vi "RF_Synth_init.vi"(1 "Initialize Instrument":u64, 2 "Inst_param":T1) -> ()   [LabVIEW 2013]
panel:
  out "Command out":string
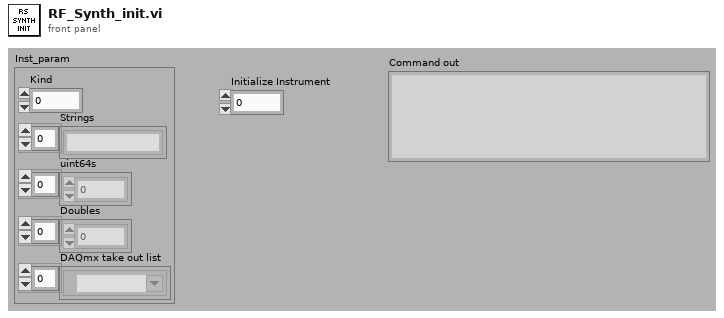
[diagram p1: front panel]
types:
  T1 = cluster{"Kind":u16, "Strings":string[], "uint64s":u64[], "Doubles":dbl[], "DAQmx take out list":refnum<k21>[]}
  T2 = enum16{"Frequency (GHz)", "Power (dBm)", "Phase (deg)", "Output on?", "Trigger mode", "Set channel", "Init"}[]
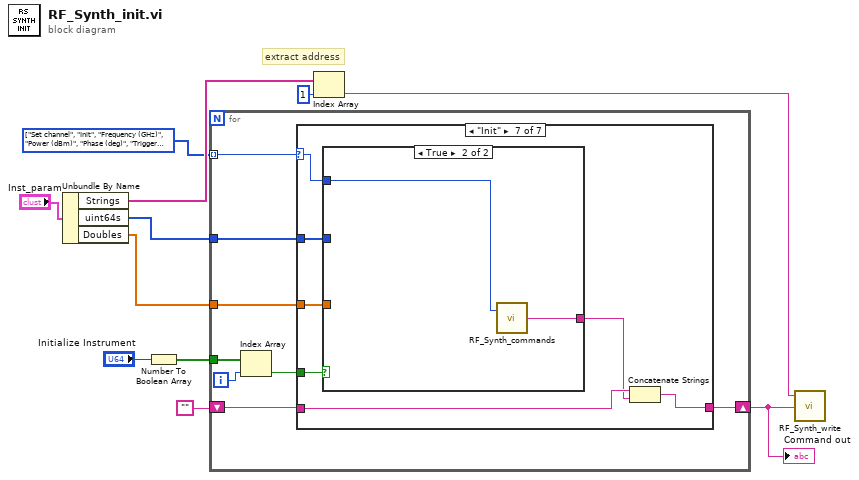
[diagram p0: block diagram]
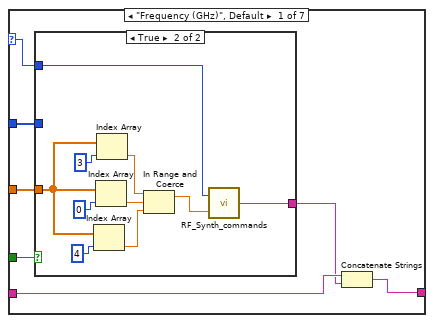
[diagram p2: hidden frame]
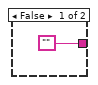
[diagram p3: hidden frame]
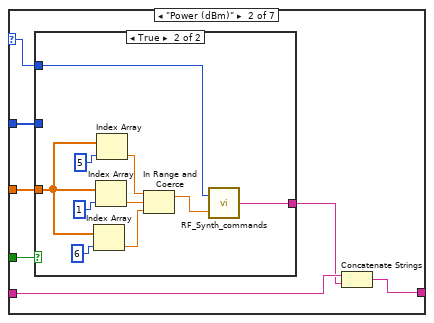
[diagram p4: hidden frame]
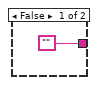
[diagram p5: hidden frame]
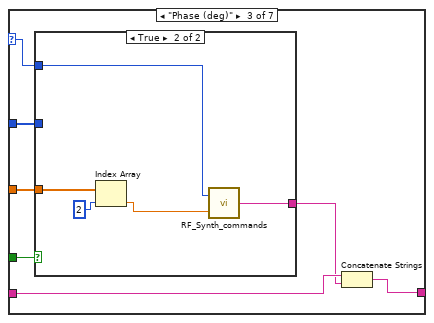
[diagram p6: hidden frame]
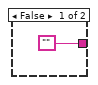
[diagram p7: hidden frame]
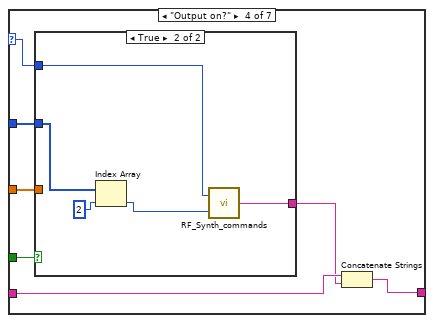
[diagram p8: hidden frame]
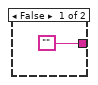
[diagram p9: hidden frame]
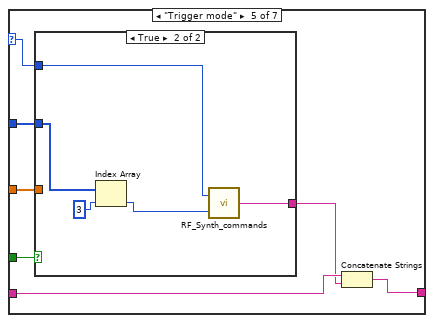
[diagram p10: hidden frame]
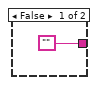
[diagram p11: hidden frame]
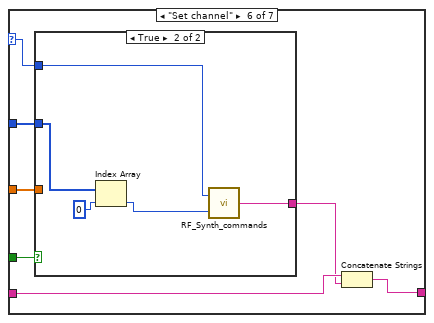
[diagram p12: hidden frame]
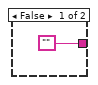
[diagram p13: hidden frame]
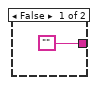
[diagram p14: hidden frame]
diagram:
  w4 = T2 [enum."Set channel", enum."Init", enum."Frequency (GHz)", enum."Power (dBm)", enum."Phase (deg)", enum."Trigger mode", enum."Output on?"] items=["Frequency (GHz)", "Power (dBm)", "Phase (deg)", "Output on?", "Trigger mode", "Set channel", "Init"]
  # "extract address"
  n1 = Unbundle By Name("Inst_param") -> ("Strings"=w10:string[], "uint64s"=w6:u64[], "Doubles"=w5:dbl[])
  n2 = Number To Boolean Array(number="Initialize Instrument") -> (Boolean array=w7:bool[])
  n3 = for {
    tunnel: w4 -> [w18] mode=indexing
    tunnel: w7 -> [w19]
    tunnel: w6 -> [w16]
    tunnel: w5 -> [w15]
    shift-right: [w13] -> w2
    shift-left: "" -> [w12]
    i -> [w14]
    n4 = Index Array(array=w19, index=w14) -> (element=w17:bool)
    n5 = case shown="\"Init\"" w18 {
      selector: w18 -> [w23 w41 w59 w72 w85 w98 w111]
      tunnel: w17 -> [w26 w44 w62 w75 w88 w101 w114]
      tunnel: w16 -> [w24 w42 w60 w73 w86 w99 w112]
      tunnel: w15 -> [w25 w43 w61 w74 w87 w100 w113]
      tunnel: w12 -> [w22 w40 w58 w71 w84 w97 w110]
      tunnel: [w21 w39 w57 w70 w83 w96 w109] -> w13
      frame "Frequency (GHz)", Default {
        n6 = case shown="True" w26 {
          tunnel: w24 -> [_ _]
          tunnel: w25 -> [_ w34]
          tunnel: w23 -> [_ w30]
          tunnel: ["" w28] -> w20
          frame False {
          }
          frame True {
            n7 = Index Array(array=w34, index=4) -> (element=w31:dbl)
            n8 = Index Array(array=w34, index=0) -> (element=w33:dbl)
            n9 = Index Array(array=w34, index=3) -> (element=w32:dbl)
            n10 = In Range and Coerce(upper limit=w32, x=w33, lower limit=w31) -> (coerced(x)=w29:dbl)  [unwired: 1 out]
            n11 = call "RF_Synth_commands.vi"("Value"=w29, "Parameter"=w30) -> ("Command"=w28:string)
          }
        }
        n12 = Concatenate Strings(w22, w20) -> (w21:string)
      }
      frame "Power (dBm)" {
        n13 = case shown="True" w44 {
          tunnel: w42 -> [_ _]
          tunnel: w43 -> [_ w52]
          tunnel: w41 -> [_ w48]
          tunnel: ["" w46] -> w38
          frame False {
          }
          frame True {
            n14 = Index Array(array=w52, index=6) -> (element=w49:dbl)
            n15 = Index Array(array=w52, index=1) -> (element=w51:dbl)
            n16 = Index Array(array=w52, index=5) -> (element=w50:dbl)
            n17 = In Range and Coerce(upper limit=w50, x=w51, lower limit=w49) -> (coerced(x)=w47:dbl)  [unwired: 1 out]
            n18 = call "RF_Synth_commands.vi"("Value"=w47, "Parameter"=w48) -> ("Command"=w46:string)
          }
        }
        n19 = Concatenate Strings(w40, w38) -> (w39:string)
      }
      frame "Phase (deg)" {
        n20 = case shown="True" w62 {
          tunnel: w60 -> [_ _]
          tunnel: w61 -> [_ w65]
          tunnel: w59 -> [_ w67]
          tunnel: ["" w66] -> w56
          frame False {
          }
          frame True {
            n21 = Index Array(array=w65, index=2) -> (element=w64:dbl)
            n22 = call "RF_Synth_commands.vi"("Value"=w64, "Parameter"=w67) -> ("Command"=w66:string)
          }
        }
        n23 = Concatenate Strings(w58, w56) -> (w57:string)
      }
      frame "Output on?" {
        n24 = case shown="True" w75 {
          tunnel: w73 -> [_ w77]
          tunnel: w74 -> [_ _]
          tunnel: w72 -> [_ w80]
          tunnel: ["" w79] -> w69
          frame False {
          }
          frame True {
            n25 = Index Array(array=w77, index=2) -> (element=w78:u64)
            n26 = call "RF_Synth_commands.vi"("Value"=w78, "Parameter"=w80) -> ("Command"=w79:string)
          }
        }
        n27 = Concatenate Strings(w71, w69) -> (w70:string)
      }
      frame "Trigger mode" {
        n28 = case shown="True" w88 {
          tunnel: w86 -> [_ w90]
          tunnel: w87 -> [_ _]
          tunnel: w85 -> [_ w93]
          tunnel: ["" w92] -> w82
          frame False {
          }
          frame True {
            n29 = Index Array(array=w90, index=3) -> (element=w91:u64)
            n30 = call "RF_Synth_commands.vi"("Value"=w91, "Parameter"=w93) -> ("Command"=w92:string)
          }
        }
        n31 = Concatenate Strings(w84, w82) -> (w83:string)
      }
      frame "Set channel" {
        n32 = case shown="True" w101 {
          tunnel: w99 -> [_ w103]
          tunnel: w100 -> [_ _]
          tunnel: w98 -> [_ w106]
          tunnel: ["" w105] -> w95
          frame False {
          }
          frame True {
            n33 = Index Array(array=w103, index=0) -> (element=w104:u64)
            n34 = call "RF_Synth_commands.vi"("Value"=w104, "Parameter"=w106) -> ("Command"=w105:string)
          }
        }
        n35 = Concatenate Strings(w97, w95) -> (w96:string)
      }
      frame "Init" {
        n36 = case shown="True" w114 {
          tunnel: w112 -> [_ _]
          tunnel: w113 -> [_ _]
          tunnel: w111 -> [_ w117]
          tunnel: ["" w116] -> w108
          frame False {
          }
          frame True {
            n37 = call "RF_Synth_commands.vi"("Parameter"=w117) -> ("Command"=w116:string)  [unwired: 1 in]
          }
        }
        n38 = Concatenate Strings(w110, w108) -> (w109:string)
      }
    }
  }
  "Command out" <- w2
  n39 = Index Array(array=w10, index=1) -> (element=w1:string)
  n40 = call "RF_Synth_write.vi"("write buffer"=w2, "VISA resource name"=w1) -> ()  [unwired: 1 in, 1 out]
